vi "printDaqDevice.vi"(8 "error in":errorcluster, 9 "Indent":i32, 10 "TreeRef":refnum<vi>, 11 "baseObject in":refnum<class "IBaseObject.lvclass">) -> (0 "error out":errorcluster, 3 "baseObject out":refnum<class "IBaseObject.lvclass">)   [LabVIEW 2022 SP3, in "openDAQ.lvlib" / "daqUtils.lvlib" / "Tree.lvlib"]
uses:
  Tree.lvlib
  IDevice/IDevice.lvclass
  IFolder/IFolder.lvclass
  ISyncComponent/ISyncComponent.lvclass
  IFunctionBlock/IFunctionBlock.lvclass
  IServer/IServer.lvclass
  IBaseObject/IBaseObject.lvclass
  IComponent/IComponent.lvclass
  IBaseObject/Polymorphic/queryInterface/queryDeviceInterface.vi
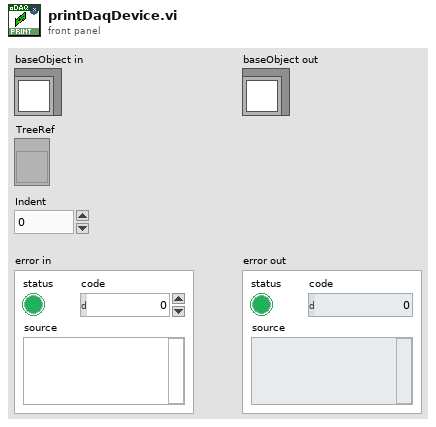
[diagram p1: front panel]
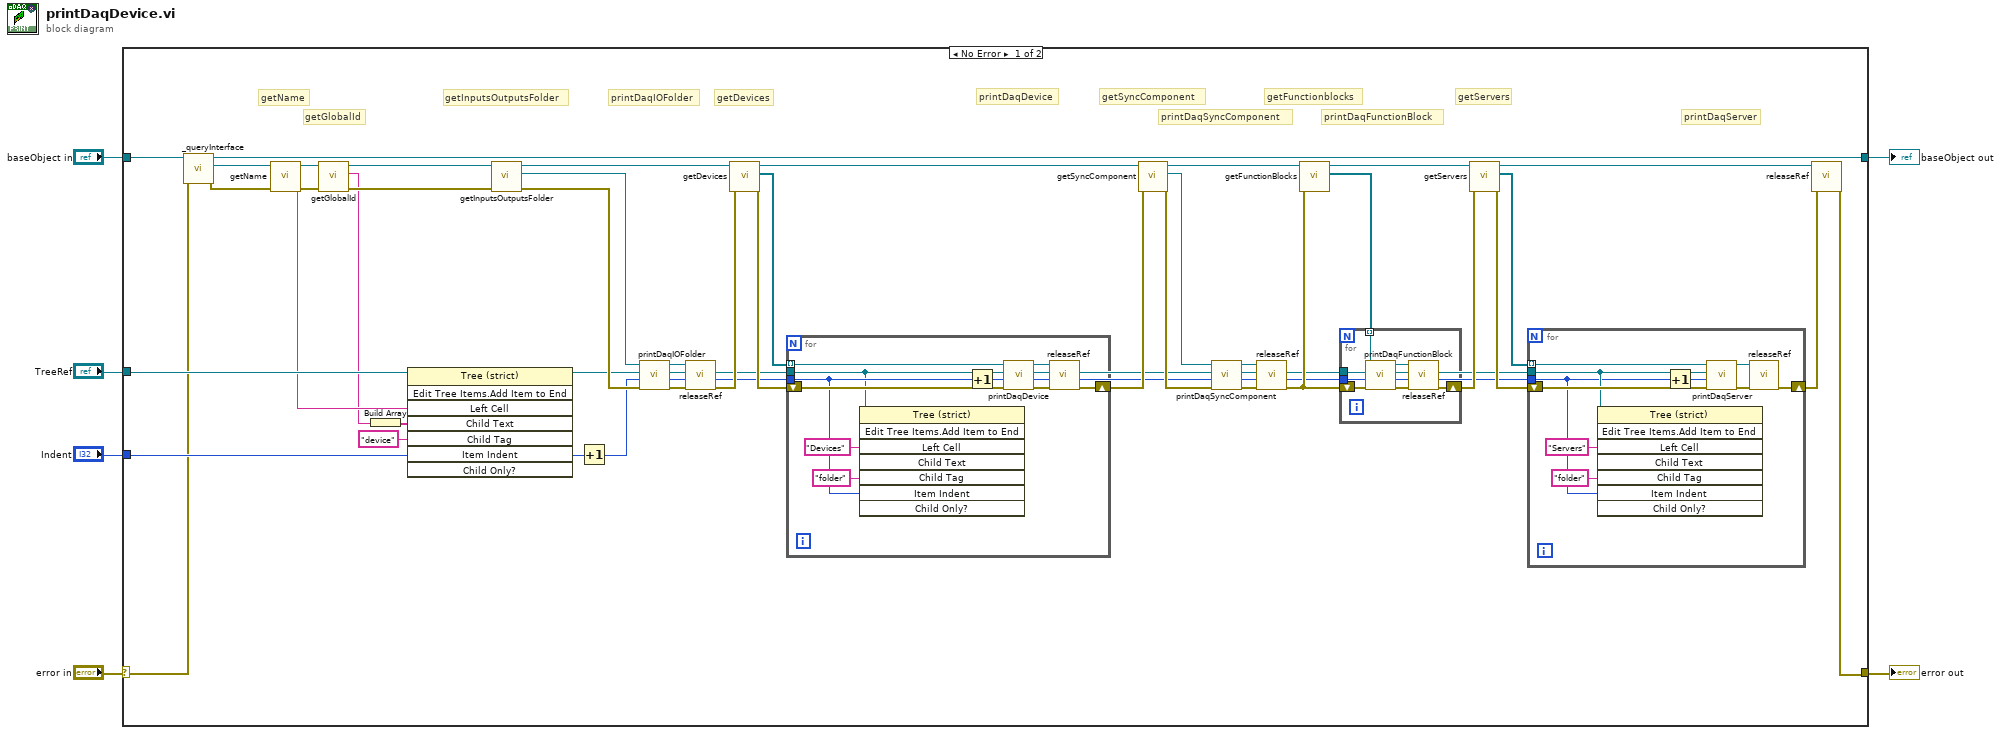
[diagram p0: block diagram]
diagram:
  n1 = case shown="No Error" "error in" {
    selector: "error in" -> [w25 w73]
    tunnel: "baseObject in" -> [w44 w72]
    tunnel: "Indent" -> [w41 _]
    tunnel: "TreeRef" -> [w27 _]
    tunnel: [w42 w73] -> w2
    tunnel: [w43 w72] -> w1
    frame No Error {
      # "printDaqServer"
      # "getServers"
      # "printDaqFunctionBlock"
      # "getFunctionblocks"
      # "printDaqSyncComponent"
      # "getSyncComponent"
      # "printDaqDevice"
      # "getDevices"
      # "printDaqIOFolder"
      # "getInputsOutputsFolder"
      # "getGlobalId"
      # "getName"
      n2 = call-poly "_queryInterface.vi"("error in (no error)"=w25, "IBaseObject in"=w44) -> ("error out"=w11:errorcluster, "IDevice out"=w13:refnum<class "IDevice.lvclass">, "IBaseObject out"=w43:refnum<class "IBaseObject.lvclass">)  [unwired: 7 in]
      n3 = call "getName.vi"("error in (no error)"=w11, "IComponent in"=w13) -> ("error out"=w10:errorcluster, "Name out"=w9:string, "IComponent out"=w12:refnum<class "IDevice.lvclass">)  [unwired: 7 in]
      n4 = call "getGlobalId.vi"("error in (no error)"=w10, "IComponent in"=w12) -> ("error out"=w45:errorcluster, "GlobalId out"=w8:string, "IComponent out"=w32:refnum<class "IDevice.lvclass">)  [unwired: 7 in]
      n5 = Build Array(w8) -> (w7:string[])
      n6 = invoke class="Tree (strict)" method="Edit Tree Items.Add Item to End"(reference=w27, "Left Cell"=w9, "Child Text"=w7, "Child Tag"="device", "Item Indent"=w41) -> (reference out=w16:refnum<vi>)  [unwired: 3 in, 7 out]
      n7 = call "getInputsOutputsFolder.vi"("error in (no error)"=w45, "IDevice in"=w32) -> ("error out"=w36:errorcluster, "IFolder out"=w35:refnum<class "IFolder.lvclass">, "IDevice out"=w30:refnum<class "IDevice.lvclass">)  [unwired: 7 in]
      n8 = Increment(x=w41) -> (x+1=w15:i32)
      n9 = call "printDaqIOFolder.vi"("Indent"=w15, "TreeRef"=w16, "baseObject in"=w35) -> ("baseObject out"=w33:refnum<class "IFolder.lvclass">)  [unwired: 7 in, 1 out]
      n10 = call-dynamic "releaseRef.vi"("error in (no error)"=w36, "IBaseObject in"=w33) -> ("error out"=w31:errorcluster)  [unwired: 9 in]
      n11 = call "getDevices.vi"("error in (no error)"=w31, "IDevice in"=w30) -> ("error out"=w38:errorcluster, "Available Devices out"=w37:refnum<class "IDevice.lvclass">[], "IDevice out"=w28:refnum<class "IDevice.lvclass">)  [unwired: 7 in]
      n12 = for {
        tunnel: w37 -> [w52] mode=indexing
        shift-right: [w53] -> w29
        shift-left: w38 -> [w54]
        tunnel: w16 -> [w47]
        tunnel: w15 -> [w46]
        n13 = invoke class="Tree (strict)" method="Edit Tree Items.Add Item to End"(reference=w47, "Left Cell"="Devices" ("Left Cell String"), "Child Tag"="folder", "Item Indent"=w46) -> ()  [unwired: 4 in, 8 out]
        n14 = Increment(x=w46) -> (x+1=w49:i32)
        n15 = call "printDaqDevice.vi"("Indent"=w49, "TreeRef"=w47, "baseObject in"=w52) -> ("baseObject out"=w51:refnum<class "IDevice.lvclass">)  [unwired: 7 in, 1 out]
        n16 = call-dynamic "releaseRef.vi"("error in (no error)"=w54, "IBaseObject in"=w51) -> ("error out"=w53:errorcluster)  [unwired: 9 in]
      }
      n17 = call "getSyncComponent.vi"("error in (no error)"=w29, "IDevice in"=w28) -> ("error out"=w40:errorcluster, "SyncComponent out"=w39:refnum<class "ISyncComponent.lvclass">, "IDevice out"=w24:refnum<class "IDevice.lvclass">)  [unwired: 7 in]
      n18 = call "printDaqSyncComponent.vi"("Indent"=w15, "TreeRef"=w16, "baseObject in"=w39) -> ("baseObject out"=w34:refnum<class "ISyncComponent.lvclass">)  [unwired: 7 in, 1 out]
      n19 = call-dynamic "releaseRef.vi"("error in (no error)"=w40, "IBaseObject in"=w34) -> ("error out"=w21:errorcluster)  [unwired: 9 in]
      n20 = call "getFunctionBlocks.vi"("error in (no error)"=w21, "IDevice in"=w24) -> ("Available Signals out"=w20:refnum<class "IFunctionBlock.lvclass">[], "IDevice out"=w23:refnum<class "IDevice.lvclass">)  [unwired: 7 in, 1 out]
      n21 = for {
        shift-right: [w65] -> w19
        shift-left: w21 -> [w71]
        tunnel: w20 -> [w70] mode=indexing
        tunnel: w16 -> [w69]
        tunnel: w15 -> [w68]
        n22 = call "printDaqFunctionBlock.vi"("error in"=w71, "Indent"=w68, "TreeRef"=w69, "baseObject in"=w70) -> ("error out"=w67:errorcluster, "baseObject out"=w66:refnum<class "IFunctionBlock.lvclass">)  [unwired: 6 in]
        n23 = call-dynamic "releaseRef.vi"("error in (no error)"=w67, "IBaseObject in"=w66) -> ("error out"=w65:errorcluster)  [unwired: 9 in]
      }
      n24 = call "getServers.vi"("error in (no error)"=w19, "IDevice in"=w23) -> ("error out"=w18:errorcluster, "Available Signals out"=w17:refnum<class "IServer.lvclass">[], "IDevice out"=w22:refnum<class "IDevice.lvclass">)  [unwired: 7 in]
      n25 = for {
        shift-right: [w60] -> w14
        shift-left: w18 -> [w64]
        tunnel: w17 -> [w63] mode=indexing
        tunnel: w16 -> [w57]
        tunnel: w15 -> [w55]
        n26 = invoke class="Tree (strict)" method="Edit Tree Items.Add Item to End"(reference=w57, "Left Cell"="Servers" ("Left Cell String"), "Child Tag"="folder", "Item Indent"=w55) -> ()  [unwired: 4 in, 8 out]
        n27 = Increment(x=w55) -> (x+1=w56:i32)
        n28 = call "printDaqServer.vi"("error in"=w64, "Indent"=w56, "TreeRef"=w57, "baseObject in"=w63) -> ("error out"=w62:errorcluster, "baseObject out"=w61:refnum<class "IServer.lvclass">)  [unwired: 6 in]
        n29 = call-dynamic "releaseRef.vi"("error in (no error)"=w62, "IBaseObject in"=w61) -> ("error out"=w60:errorcluster)  [unwired: 9 in]
      }
      n30 = call-dynamic "releaseRef.vi"("error in (no error)"=w14, "IBaseObject in"=w22) -> ("error out"=w42:errorcluster)  [unwired: 9 in]
    }
    frame Error {
    }
  }
  "error out" <- w2
  "baseObject out" <- w1
